vi "etc_XCITE_GetVersion.vi"(0 "h":u64, 5 "error in (no error)":errorcluster {"code" format="%x"}) -> (13 "build":i32, 14 "h out":u64, 15 "ErrorMessage":i32 format="%x", 16 "major":i32, 17 "minor":i32, 18 "patch":i32, 19 "error out":errorcluster {"code" format="%x"})   [LabVIEW 2019, in "XCite.lvlib"]
doc: "Get information about the X-cite device firmware"
uses:
  XCite.lvlib
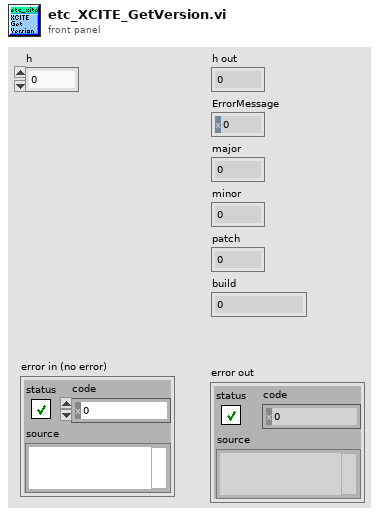
[diagram p1: front panel]
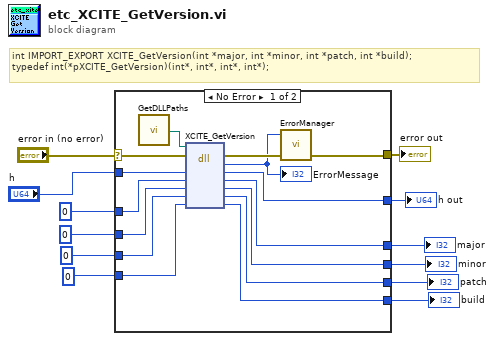
[diagram p0: block diagram]
diagram:
  # "int IMPORT_EXPORT XCITE_GetVersion(int *major, int *minor, int *patch, int *build);\ntypedef int(*pXCITE_GetVersion)(int*, int*, int*, int*);"
  n1 = case shown="No Error" "error in (no error)" {
    selector: "error in (no error)" -> [w27 w33]
    tunnel: [w25 w33] -> w12
    tunnel: "h" -> [w23 w32]
    tunnel: [w22 w32] -> w10
    tunnel: 0 ("open_count") -> [w20 w28]
    tunnel: [w19 w31] -> w7
    tunnel: 0 ("major") -> [w18 w31]
    tunnel: 0 ("minor") -> [w17 w30]
    tunnel: 0 ("patch") -> [w16 w29]
    tunnel: [w15 w30] -> w3
    tunnel: [w14 w29] -> w2
    tunnel: [w13 w28] -> w1
    frame No Error {
      n2 = call "GetDLLPaths.vi"() -> ("etc_xcite_path"=w21:path)  [unwired: 8 in, 3 out]
      n3 = dll-call lib="?" fn="XCITE_GetVersion"(path in=w21, error in=w27, "h"=w23, "major"=w18, "minor"=w17, "patch"=w16, "build"=w20) -> (error out=w26:errorcluster, "return type"=w24:i32, "h"=w22:u64, "major"=w19:i32, "minor"=w15:i32, "patch"=w14:i32, "build"=w13:i32)  [unwired: 1 in, 1 out]
      "ErrorMessage" <- w24
      n4 = call "ErrorManager.vi"("error in (no error)"=w26, "error code"=w24) -> ("error out"=w25:errorcluster)  [unwired: 2 in, 1 out]
    }
    frame Error {
    }
  }
  "error out" <- w12
  "h out" <- w10
  "build" <- w1
  "major" <- w7
  "minor" <- w3
  "patch" <- w2
